vi "Write Google Earth KML File.vi"() -> ()   [LabVIEW 2011]
uses:
  <vilib>/Platform/browser.llb/Open URL in Default Browser (path).vi
panel:
  in  "kml":T1={"#attributes"={"xmlns"="http://earth.google.com/kml/2.0"}, "Document"={"Placemark"=[{"name"="New York", "Point"={"coordinates"="-74.00639,40.71417"}}, {"name"="Austin", "Point"={"coordinates"="-97.74278,30.26694"}}, {"name"="San Francisco", "Point"={"coordinates"="-122.41833,37.775"}}]}}
  # "Run this VI to write the 'Playlist' cluster (left) to an XML File and then read the data and format back into 'Playlist Out' cluster (right)"
  # "Run this VI to create a KML file from the structure below and open it in Google Earth.\nGet Google Earth from http://earth.google.com"
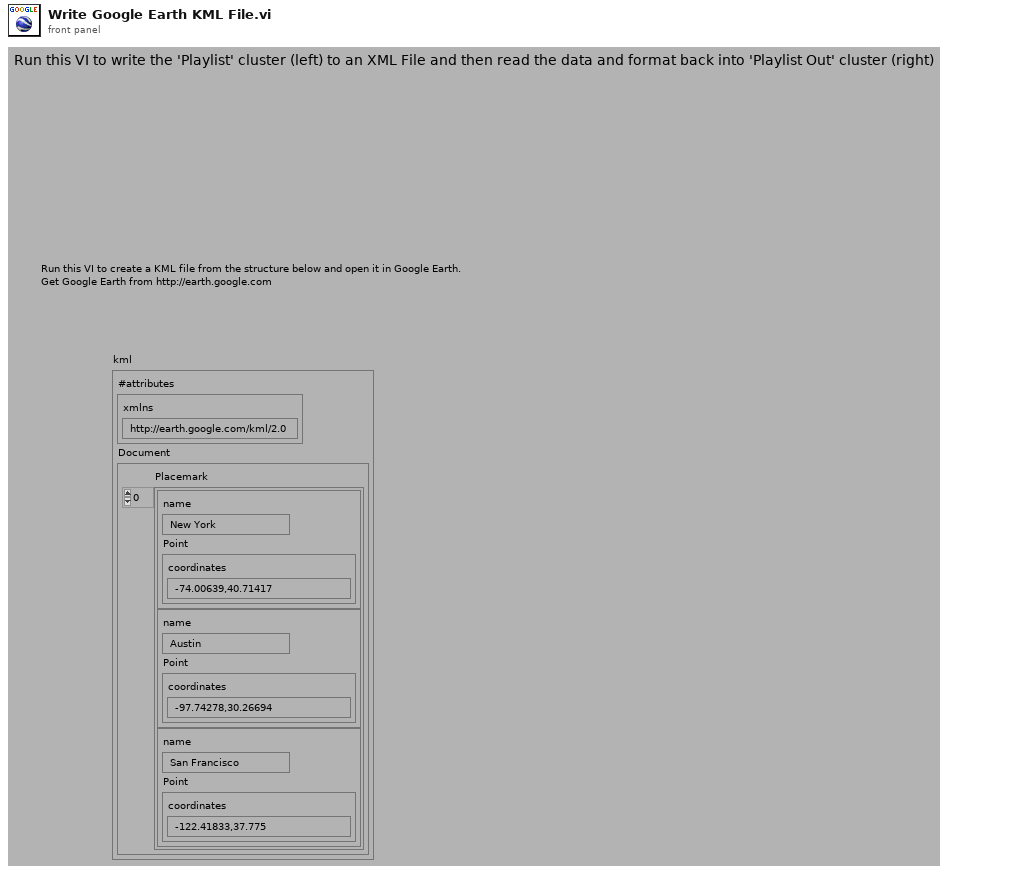
[diagram p1: front panel]
types:
  T1 = cluster{"#attributes":cluster{"xmlns":string}, "Document":cluster{"Placemark":cluster{"name":string, "Point":cluster{"coordinates":string}}[]}}
  T2 = enum32{"existing file", "new file", "new or existing file", "existing dir", "new dir", "new or existing dir", "existing file (use LLBs)", "new file (use LLBs)", "new or existing file (use LLBs)", "new or existing file or directory (use LLBs)"}
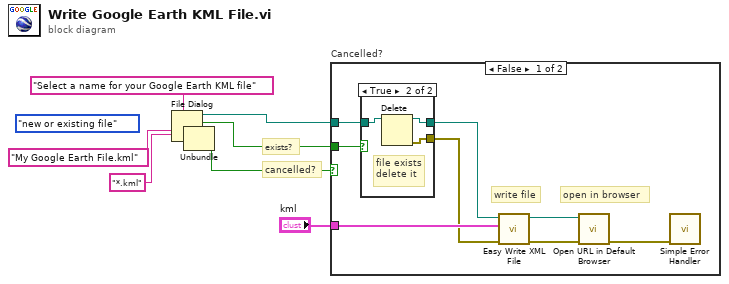
[diagram p0: block diagram]
diagram:
  (unwired) T2."new or existing file" ("select mode (2)")
  # "exists?"
  # "cancelled?"
  n1 = File Dialog(6:"*.kml" ("pattern"), 7:"Select a name for your Google Earth KML file" ("prompt"), 9:"My Google Earth File.kml" ("default name")) -> (0:w1:errorcluster, 1:w2:bool, 2:w4:bool, 3:w3:path)  [unwired: 4 in]
  n2 = Unbundle(w1) -> ()  [unwired: 3 out]
  n3 = case "Cancelled?" shown="False" w2 {
    tunnel: "kml" -> [w16 _]
    tunnel: w4 -> [w15 _]
    tunnel: w3 -> [w14 _]
    frame False {
      # "open in browser"
      # "write file"
      n4 = case shown="True" w15 {
        tunnel: w14 -> [w17 w20]
        tunnel: [w17 w19] -> w12
        tunnel: [_ w18] -> w13
        frame False {
        }
        frame True {
          # "file exists\ndelete it"
          n5 = Delete(path (use dialog)=w20) -> (deleted path=w19:path, error out=w18:errorcluster)  [unwired: 4 in, 1 out]
        }
      }
      n6 = call "Easy Write XML File.vi"("error in (no error)"=w13, "LabVIEW Data"=w16, "XML File Path"=w12) -> ("error out"=w11:errorcluster, "XML File Path (duplicate)"=w9:path)  [unwired: 7 in]
      n7 = call-poly <vilib>:"Open URL in Default Browser.vi"("error in (no error)"=w11, "path"=w9) -> ("error out"=w10:errorcluster)  [unwired: 4 in, 1 out]
      n8 = call <vilib>:"Simple Error Handler.vi"("error in (no error)"=w10) -> ()  [unwired: 4 in, 5 out]
    }
    frame True {
    }
  }
